vi "Delay Time.vi"(10 "error in (no error)":errorcluster, 11 "Delay(ms)":u32=30) -> (2 "error out":errorcluster)   [LabVIEW 2015]
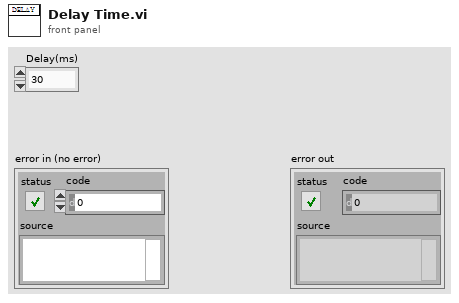
[diagram p1: front panel]
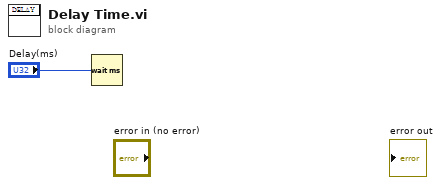
[diagram p0: block diagram]
diagram:
  n1 = Wait (ms)(milliseconds to wait="Delay(ms)") -> ()  [unwired: 1 out]
